vi "Init HTTP Server.vi"(8 "error in (no error)":errorcluster, 11 "VideoMux in":refnum<class "VideoMux.lvclass">) -> (0 "error out":errorcluster, 3 "VideoMux out":refnum<class "VideoMux.lvclass">)   [LabVIEW 2022 SP3, in "VideoMux.lvlib" / "VideoMux.lvclass"]
uses:
  VideoMux.lvclass
  CurrentStateController/CurrentStateController.lvclass
  C:/Program Files (x86)/National Instruments/LabVIEW 2022/vi.lib/IlluminatedG/IG HTTP Server/HTTP Server/Handler/Handler.lvclass
  ConnectRouteController/ConnectRouteController.lvclass
  VideoMux.lvclass/VideoMux.ctl
  MuxAPI/MuxAPI.lvclass
  C:/Program Files (x86)/National Instruments/LabVIEW 2022/vi.lib/IlluminatedG/IG HTTP Server/HTTP Server/Service/Service.lvclass
  <vilib>/IlluminatedG/IG HTTP Server/HTTP Server/Server/Add Connection Handler.vi
  <vilib>/IlluminatedG/IG HTTP Server/HTTP Server/Server/Add Request Handler.vi
  <vilib>/IlluminatedG/IG HTTP Server/HTTP Server/Server/Add Route Handler.vi
  <vilib>/IlluminatedG/IG HTTP Server/HTTP Server/Server/Add Controller Handler.vi
  <vilib>/IlluminatedG/IG HTTP Server/HTTP Server/Server/Add Controller.vi
  <vilib>/IlluminatedG/IG HTTP Server/HTTP Server/Server/Add Response Handler.vi
  <vilib>/IlluminatedG/IG HTTP Server/HTTP Server/Server/Add Complete Handler.vi
  <vilib>/IlluminatedG/IG HTTP Server/HTTP Server/Server/Add Exception Handler.vi
  <vilib>/IlluminatedG/IG HTTP Server/HTTP Server/Connection Handler/Connection Handler.lvclass
  <vilib>/IlluminatedG/IG HTTP Server/HTTP Server/Request Handler/Request Handler.lvclass
  <vilib>/IlluminatedG/IG HTTP Server/HTTP Server/Route Handler/Route Handler.lvclass
  <vilib>/IlluminatedG/IG HTTP Server/HTTP Server/Controller Handler/Controller Handler.lvclass
  <vilib>/IlluminatedG/IG HTTP Server/HTTP Server/Controller/Controller.lvclass
  <vilib>/IlluminatedG/IG HTTP Server/HTTP Server/Response Handler/Response Handler.lvclass
  <vilib>/IlluminatedG/IG HTTP Server/HTTP Server/Complete Handler/Complete Handler.lvclass
  <vilib>/IlluminatedG/IG HTTP Server/HTTP Server/Exception Handler/Exception Handler.lvclass
  <vilib>/IlluminatedG/IG HTTP Server/HTTP Server/Handler/Handler.lvclass
  <vilib>/IlluminatedG/IG HTTP Server/HTTP Server/Server/Server.lvclass
  C:/dev/illuminatedg/TouchControl/VideoMux/MuxAPI/MuxAPI.lvclass
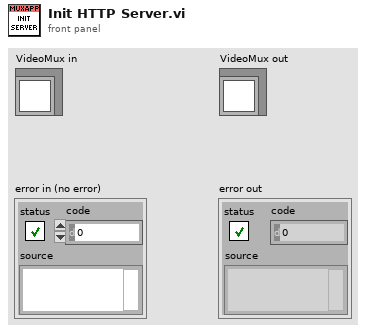
[diagram p1: front panel]
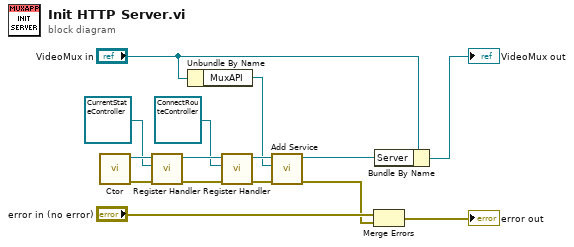
[diagram p0: block diagram]
diagram:
  n1 = call <vilib>:"Ctor.vi"() -> ("error out"=w13:errorcluster, "Server out"=w14:refnum<class "Server.lvclass">)  [unwired: 10 in]
  n2 = call <vilib>:"Register Handler.vi"("error in (no error)"=w13, "Handler"=refnum<class "CurrentStateController.lvclass"> refnum ("VideoMux.lvlib:CurrentStateController.lvclass"), "Server in"=w14) -> ("error out"=w10:errorcluster, "Server out"=w11:refnum<class "Server.lvclass">)  [unwired: 7 in]
  n3 = Unbundle By Name("VideoMux in") -> ("MuxAPI"=w6:refnum<class "MuxAPI.lvclass">)
  n4 = call <vilib>:"Register Handler.vi"("error in (no error)"=w10, "Handler"=refnum<class "ConnectRouteController.lvclass"> refnum ("VideoMux.lvlib:ConnectRouteController.lvclass"), "Server in"=w11) -> ("error out"=w7:errorcluster, "Server out"=w8:refnum<class "Server.lvclass">)  [unwired: 7 in]
  n5 = call <vilib>:"Add Service.vi"("error in (no error)"=w7, "Service"=w6, "Server in"=w8) -> ("error out"=w1:errorcluster, "Server out"=w2:refnum<class "Server.lvclass">)  [unwired: 7 in]
  n6 = Merge Errors("error in (no error)", w1) -> (→"error out":errorcluster)
  n7 = Bundle By Name(cluster="VideoMux in", "Server"=w2) -> (→"VideoMux out":refnum<class "VideoMux.lvclass">)
